vi "test1-AllChainNodesShareTheSameData.vi"(8 "error in (no error)":errorcluster, 11 "TestCase in":refnum<class "testcase-CSMChainMode.lvclass">) -> (0 "error out":errorcluster, 3 "TestCase out":refnum<class "testcase-CSMChainMode.lvclass">)   [LabVIEW 2017, in "testcase-CSMChainMode.lvclass"]
uses:
  testcase-CSMChainMode.lvclass
  src/user.lib/_NEVSTOP/Communicable State Machine(CSM)/_Support/Typedef/_CSM_MODE.ctl
  8deca385-1376-47bb-b92d-c44567c1a462.vi
  <vilib>/addons/_JKI Toolkits/VI Tester/TestCase.llb/TestCase.lvclass
  src/user.lib/_NEVSTOP/Communicable State Machine(CSM)/Communicable State Machine.lvlib
  C:/Program Files (x86)/National Instruments/LabVIEW 2017/vi.lib/addons/_JKI Toolkits/VI Tester/TestCase.llb/TestCase.lvclass
panel:
  out "error out 2":errorcluster
  out "LoopCount":i32
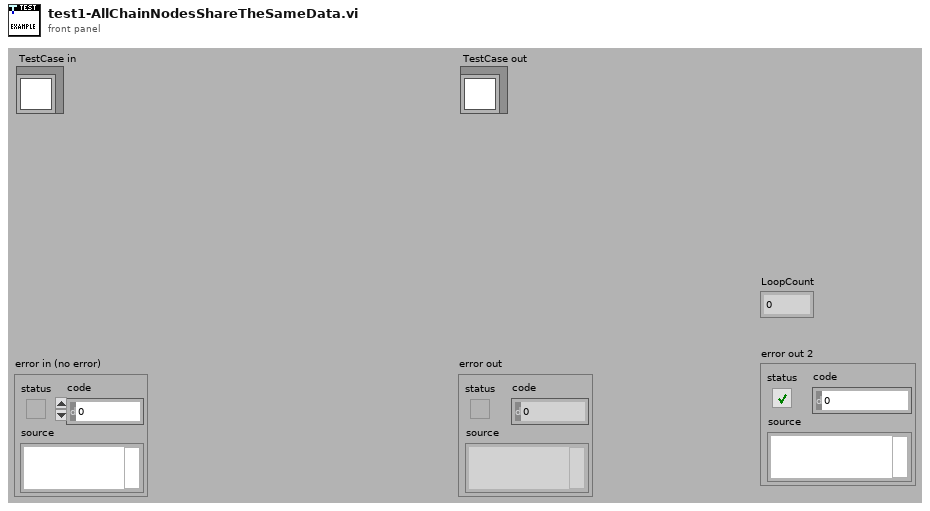
[diagram p1: front panel]
types:
  T1 = typedef "Communicable State Machine.lvlib/_CSM_MODE.ctl" = enum16{"Not Exist", "Stand Alone", "CSM", "Worker", "Worker Agent", "Chain Node", "Chain"}
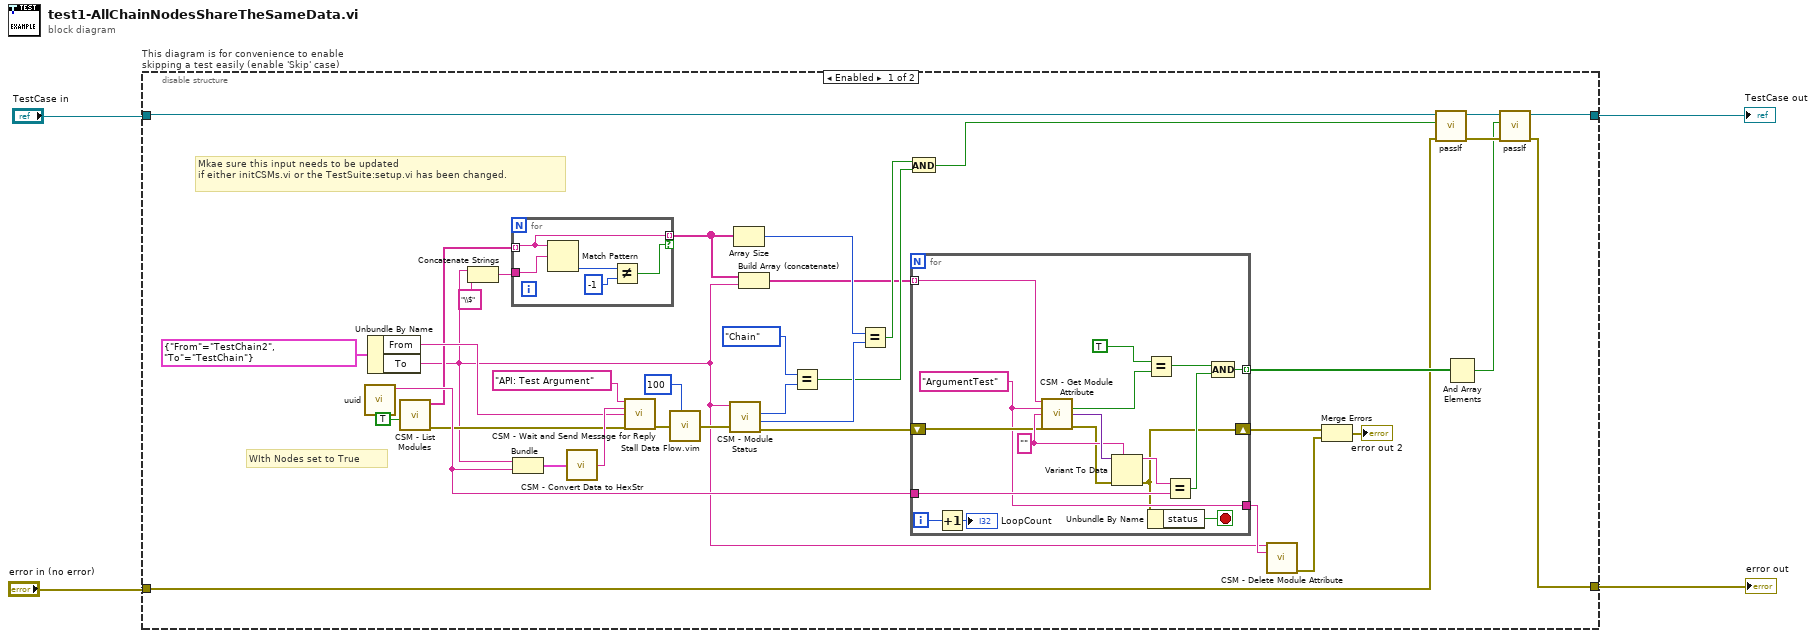
[diagram p0: block diagram]
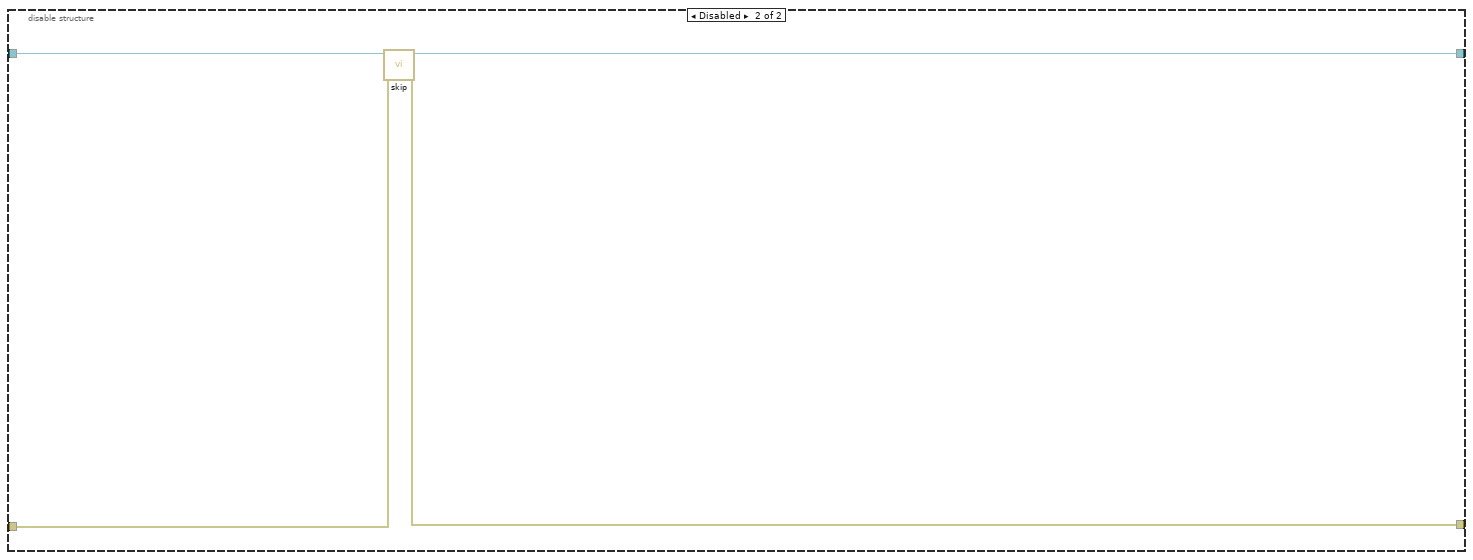
[diagram p2: hidden frame]
diagram:
  n1 = disable-structure "This diagram is for convenience to enable skipping a test easily (enable 'Skip' case)" shown="Enabled" {
    disable-tunnel: "TestCase in" -> [w11 w67]
    disable-tunnel: [w10 w65] -> w1
    disable-tunnel: [w9 w66] -> w3
    disable-tunnel: "error in (no error)" -> [w12 w64]
    frame Enabled {
      # "Mkae sure this input needs to be updated \nif either initCSMs.vi or the TestSuite:setup.vi has been changed."
      # "WIth Nodes set to True"
      n2 = call "uuid.vi"() -> ("UUID"=w35:string)  [unwired: 11 in]
      n3 = Unbundle By Name(cluster{"From":string, "To":string} {"From"="TestChain2", "To"="TestChain"} ("Cluster")) -> ("From"=w36:string, "To"=w6:string)
      n4 = call "CSM - List Modules.vi"("With Nodes? (F)"=TRUE) -> ("error out"=w29:errorcluster, "Module Names"=w32:string[])  [unwired: 9 in]
      n5 = Concatenate Strings(w6, "\\$" ("string")) -> (w7:string)
      n6 = for {
        tunnel: w32 -> [w61] mode=indexing
        tunnel: [w61] -> w21 mode=indexing if=w60
        tunnel: w7 -> [w59]
        n7 = Match Pattern(string=w61, regular expression=w59) -> (offset past match=w63:i32)  [unwired: 1 in, 3 out]
        n8 = Not Equal?(x=w63, y=-1) -> (x != y?=w60:bool)
      }
      n9 = Bundle("To"=w6, "UUID"=w35) -> (w38:cluster{"To":string, "UUID":string})  [unwired: 1 in]
      n10 = call "CSM - Convert Data to HexStr.vi"("Variant"=w38) -> ("HEX String (0-9,A-F)"=w37:string)  [unwired: 8 in]
      n11 = call "CSM - Wait and Send Message for Reply.vi"("State"="API: Test Argument", "Arguments (\"\")"=w37, "Target Module"=w36, "Error In (No Error)"=w29) -> ("error out"=w40:errorcluster)  [unwired: 8 in, 3 out]
      n12 = call "Stall Data Flow.vim"("value in"=w40, "milliseconds to wait"=u32 100) -> ("value out"=w34:errorcluster)  [unwired: 1 out]
      n13 = call "CSM - Module Status.vi"("Error In"=w34, "CSM Name"=w6) -> ("error out"=w19:errorcluster, "#Nodes"=w28:i32, "Mode"=w30:T1)  [unwired: 5 in, 2 out]
      n14 = Array Size(array=w21) -> (size(s)=w27:i32)
      n15 = Build Array (concatenate)(w21, w6) -> (w20:string[])
      n16 = Equal?(x=_CSM_MODE."Chain" ("Mode 2"), y=w30) -> (x = y?=w25:bool)
      n17 = Equal?(x=w27, y=w28) -> (x = y?=w26:bool)
      n18 = And(x=w26, y=w25) -> (x .and. y?=w24:bool)
      n19 = for {
        tunnel: w35 -> [w58]
        tunnel: w20 -> [w49] mode=indexing
        shift-right: [w43] -> w15
        shift-left: w19 -> [w48]
        tunnel: [w47] -> w18 mode=indexing
        tunnel: [w46] -> w16
        i -> [w45]
        stop <- w42 stop-if-true
        w54 = ""
        w46 = "ArgumentTest" ("Attribute")
        n20 = Increment(x=w45) -> (x+1=→"LoopCount":i32)
        n21 = call "CSM - Get Module Attribute.vi"("CSM Name"=w49, "Attribute"=w46, "Default Value (Empty Variant)"=w54, "Error In"=w48) -> ("Found"=w57:bool, "Value"=w55:variant, "error out"=w52:errorcluster)  [unwired: 7 in, 2 out]
        n22 = Variant To Data(error in=w52, type=w54, Variant=w55) -> (data=w53:string, error out=w43:errorcluster)
        n23 = Equal?(x=TRUE, y=w57) -> (x = y?=w51:bool)
        n24 = Unbundle By Name(w43) -> ("status"=w42:bool)
        n25 = Equal?(x=w53, y=w58) -> (x = y?=w50:bool)
        n26 = Compound Arithmetic op=AND(w51, w50) -> (w47:bool)
      }
      n27 = call "CSM - Delete Module Attribute.vi"("CSM Name"=w6, "Attribute"=w16) -> ("error out"=w14:errorcluster)  [unwired: 10 in, 3 out]
      n28 = Merge Errors(w15, w14) -> (→"error out 2":errorcluster)
      n29 = call-dynamic "passIf.vi"("error in (no error)"=w12, "pass"=w24, "TestCase in"=w11) -> ("error out"=w22:errorcluster, "TestCase out"=w23:refnum<class "testcase-CSMChainMode.lvclass">)  [unwired: 7 in]
      n30 = And Array Elements(Boolean array=w18) -> (logical AND=w17:bool)
      n31 = call-dynamic "passIf.vi"("error in (no error)"=w22, "pass"=w17, "TestCase in"=w23) -> ("error out"=w9:errorcluster, "TestCase out"=w10:refnum<class "testcase-CSMChainMode.lvclass">)  [unwired: 7 in]
    }
    frame Disabled {
      # "skip test result while test is under development"
      n32 = call <vilib>:"skip.vi"("error in (no error)"=w64, "TestCase in"=w67) -> ("error out"=w66:errorcluster, "TestCase out"=w65:refnum<class "testcase-CSMChainMode.lvclass">)  [unwired: 8 in]
    }
  }
  "error out" <- w3
  "TestCase out" <- w1
